vi "test Write and Read Float.vi"(8 "error in (no error)":errorcluster, 11 "TestCase in":refnum<class "Read Value Tests.lvclass">) -> (0 "error out":errorcluster, 3 "TestCase out":refnum<class "Read Value Tests.lvclass">)   [LabVIEW 2020, in "Memory Manager Tests.lvlib" / "Read Value Tests.lvclass"]
uses:
  Read Value Tests.lvclass
  Read Value Tests.lvclass/Read Value Tests.ctl
  Source/Classes/Pointer/Read SGL.vi
  Source/Classes/Pointer/Read DBL.vi
  <vilib>/addons/_JKI Toolkits/VI Tester/TestCase.llb/TestCase.lvclass
  Source/Classes/Pointer/Pointer.lvclass
  C:/Program Files (x86)/National Instruments/LabVIEW 2020/vi.lib/addons/_JKI Toolkits/VI Tester/TestCase.llb/TestCase.lvclass
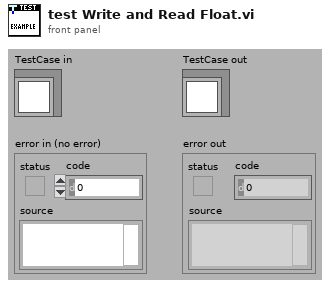
[diagram p1: front panel]
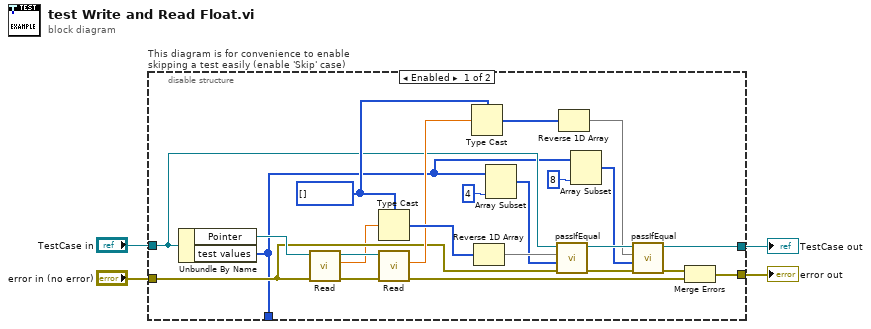
[diagram p0: block diagram]
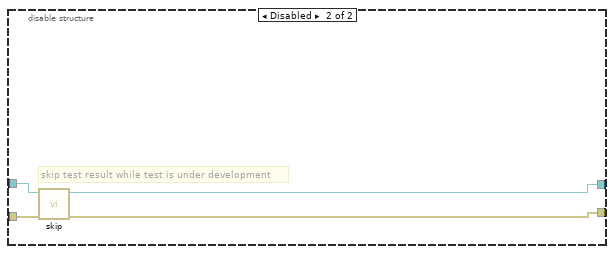
[diagram p2: hidden frame]
diagram:
  n1 = disable-structure "This diagram is for convenience to enable skipping a test easily (enable 'Skip' case)" shown="Enabled" {
    disable-tunnel: "TestCase in" -> [w11 w31]
    disable-tunnel: [w15 w29] -> w1
    disable-tunnel: [w8 w30] -> w3
    disable-tunnel: "error in (no error)" -> [w9 w28]
    disable-tunnel: [w6 _] -> _
    frame Enabled {
      w16 = u8[] [] ("buffer in")
      n2 = Unbundle By Name(w11) -> ("Pointer"=w10:refnum<class "Pointer.lvclass">, "test values"=w6:u8[])
      n3 = call-poly "Read.vi"("error in (no error)"=w9, "Pointer in"=w10) -> ("error out"=w17:errorcluster, "value out"=w5:sgl, "Pointer out"=w22:refnum<class "Pointer.lvclass">)  [unwired: 6 in, 1 out]
      n4 = Type Cast(type=w16, x=w5) -> (*(type *) &x=w27:u8[])
      n5 = call-poly "Read.vi"("error in (no error)"=w17, "Pointer in"=w22) -> ("error out"=w7:errorcluster, "value out"=w19:dbl)  [unwired: 6 in, 2 out]
      n6 = Type Cast(type=w16, x=w19) -> (*(type *) &x=w20:u8[])
      n7 = Reverse 1D Array(array=w27) -> (reversed array=w25:u8[])
      n8 = Array Subset(array=w6, length=4) -> (w13:u8[])  [unwired: 1 in]
      n9 = call-dynamic "passIfEqual.vi"("error in (no error)"=w9, "y"=w13, "x"=w25, "TestCase in"=w11) -> ("error out"=w26:errorcluster, "TestCase out"=w23:refnum<class "Read Value Tests.lvclass">)  [unwired: 6 in]
      n10 = Reverse 1D Array(array=w20) -> (reversed array=w18:u8[])
      n11 = Array Subset(array=w6, length=8) -> (w12:u8[])  [unwired: 1 in]
      n12 = call-dynamic "passIfEqual.vi"("error in (no error)"=w26, "y"=w12, "x"=w18, "TestCase in"=w23) -> ("error out"=w14:errorcluster, "TestCase out"=w15:refnum<class "Read Value Tests.lvclass">)  [unwired: 6 in]
      n13 = Merge Errors(w14, w7) -> (w8:errorcluster)
    }
    frame Disabled {
      # "skip test result while test is under development"
      n14 = call <vilib>:"skip.vi"("error in (no error)"=w28, "TestCase in"=w31) -> ("error out"=w30:errorcluster, "TestCase out"=w29:refnum<class "Read Value Tests.lvclass">)  [unwired: 8 in]
    }
  }
  "error out" <- w3
  "TestCase out" <- w1
